vi "NI VeriStand - Close Command Line Notification (Macro Player).vi"(8 "error in (no error)":errorcluster, 11 "CommandLine Refs":T1) -> (0 "error out":errorcluster)   [LabVIEW 2020, in "NI_VS MacroPlayerAPI.lvlib"]
doc: "Closes an open reference to the command line of the Macro Player tool. Use the Open Command Line Notification (Macro Player) VI to open the reference this VI closes."
uses:
  <vilib>/NI VeriStand/Execution/MacroPlayer/NI_VS MacroPlayerAPI.lvlib
  <vilib>/NI VeriStand/Execution/MacroPlayer/CommandLine Refs.ctl
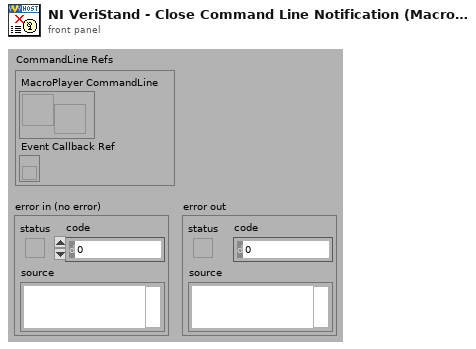
[diagram p1: front panel]
types:
  T1 = typedef "NI_VS MacroPlayerAPI.lvlib/CommandLine Refs.ctl" = cluster{"MacroPlayer CommandLine":refnum<user-event>, "Event Callback Ref":refnum<k27>}
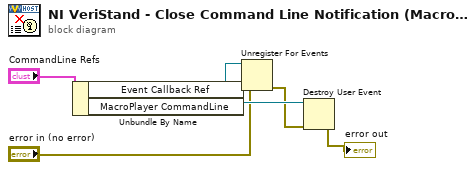
[diagram p0: block diagram]
diagram:
  n1 = Unbundle By Name("CommandLine Refs") -> ("Event Callback Ref"=w6:refnum<k27>, "MacroPlayer CommandLine"=w5:refnum<user-event>)
  n2 = Unregister For Events(event registration refnum=w6, error in="error in (no error)") -> (error out=w4:errorcluster)
  n3 = Destroy User Event(user event=w5, error in=w4) -> (error out=→"error out":errorcluster)
